vi "dbl to str.vi"(11 "Numeric":cdb) -> (3 "String":string)   [LabVIEW 2020]
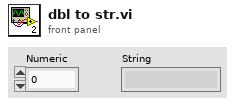
[diagram p1: front panel]
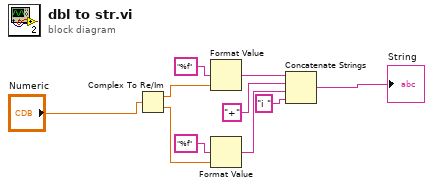
[diagram p0: block diagram]
diagram:
  n1 = Complex To Re/Im(x + iy="Numeric") -> (x=w8:dbl, y=w9:dbl)
  n2 = Format Value(format string="%f", value (0)=w8) -> (output string=w1:string)  [unwired: 1 in]
  n3 = Format Value(format string="%f", value (0)=w9) -> (output string=w2:string)  [unwired: 1 in]
  n4 = Concatenate Strings(w1, "+" ("string"), w2, "i " ("string")) -> (→"String":string)
